vi "CTI_AOTF_GrabChannelFromGlobalVars.vi"(8 "error in":errorcluster) -> (0 "AOTF_LaserChannelWavelength":i32[](array[numeric]), 1 "AOTF_LaserChannelFixedwavelength":string[](array[string]), 2 "AOTF_LaserChannelPower":i16[](array[numeric]), 3 "AOTF_LaserChannelOnOff":bool[](array[boolean]), 4 "error out":errorcluster)   [LabVIEW 2011]
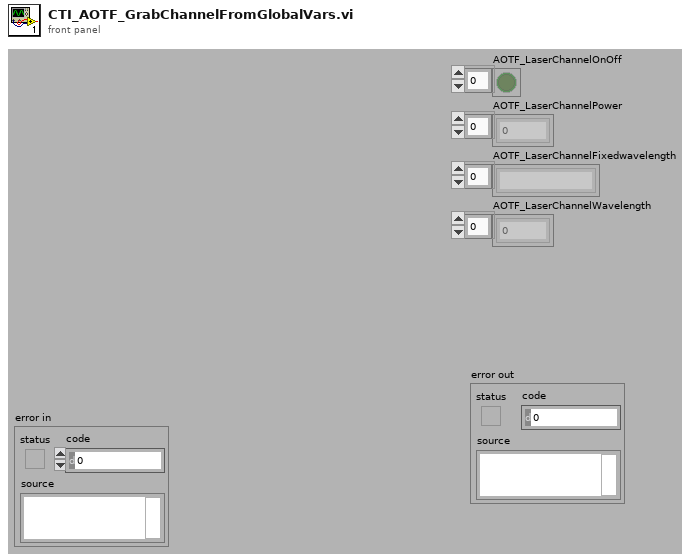
[diagram p1: front panel]
types:
  T1 = cluster{"1.LaserChannel ON/OFF":bool, "1.Laser Channel Power / [%]":i16, "1.Laser Channel Fixedwavelength":string, "1.Laser Channel Wavelength":i32, "Wavelength":enum16{"Fixed", "UserDefined"}}
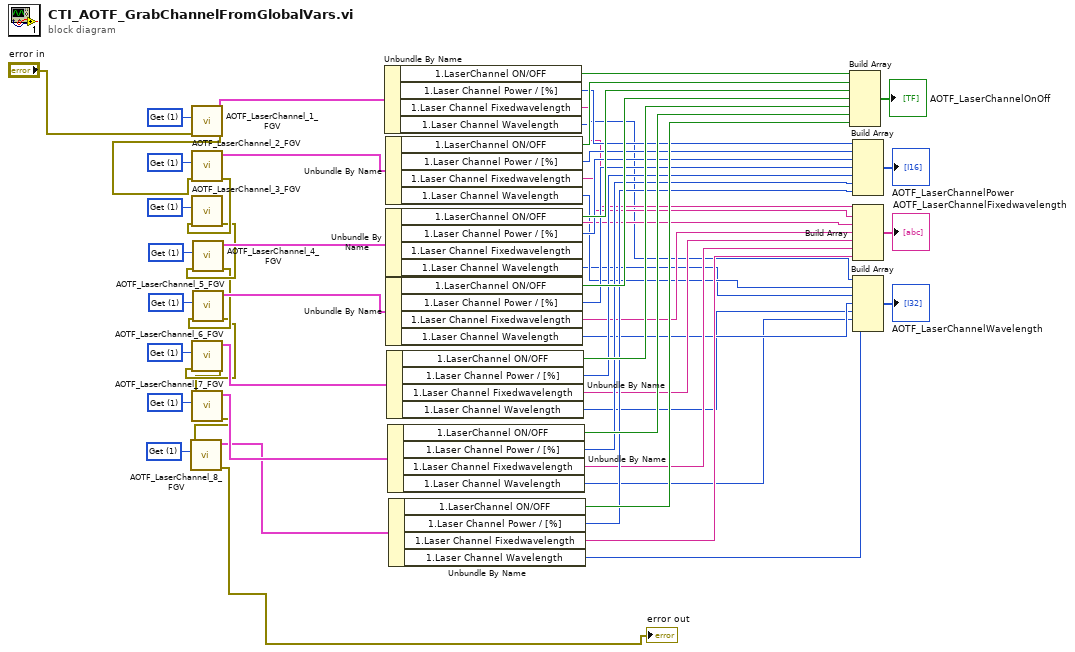
[diagram p0: block diagram]
diagram:
  w49 = u16 1 items=["Set", "Get"] ("Set_Get")
  w50 = u16 1 items=["Set", "Get"] ("Set_Get")
  w51 = u16 1 items=["Set", "Get"] ("Set_Get")
  w52 = u16 1 items=["Set", "Get"] ("Set_Get")
  w53 = u16 1 items=["Set", "Get"] ("Set_Get")
  w54 = u16 1 items=["Set", "Get"] ("Set_Get")
  w55 = u16 1 items=["Set", "Get"] ("Set_Get")
  w56 = u16 1 items=["Set", "Get"] ("Set_Get")
  n1 = call "AOTF_LaserChannel_1_FGV.vi"("error in"="error in", "Set_Get"=w56) -> ("error out"=w8:errorcluster, "LaserChannel_2_OUT"=w48:T1)  [unwired: 8 in]
  n2 = call "AOTF_LaserChannel_2_FGV.vi"("error in"=w8, "FGV_Control"=w55) -> ("error out"=w7:errorcluster, "LaserChannel_2_OUT"=w47:T1)  [unwired: 8 in]
  n3 = call "AOTF_LaserChannel_3_FGV.vi"("error in"=w7, "Set_Get"=w54) -> ("error out"=w6:errorcluster)  [unwired: 8 in, 1 out]
  n4 = call "AOTF_LaserChannel_4_FGV.vi"("error in"=w6, "Set_Get"=w53) -> ("error out"=w5:errorcluster, "LaserChannel_2_OUT"=w46:T1)  [unwired: 8 in]
  n5 = call "AOTF_LaserChannel_5_FGV.vi"("error in"=w5, "Set_Get"=w52) -> ("error out"=w4:errorcluster, "LaserChannel_2_OUT"=w45:T1)  [unwired: 8 in]
  n6 = call "AOTF_LaserChannel_6_FGV.vi"("error in"=w4, "Set_Get"=w51) -> ("error out"=w3:errorcluster, "LaserChannel_2_OUT"=w44:T1)  [unwired: 8 in]
  n7 = call "AOTF_LaserChannel_7_FGV.vi"("error in"=w3, "Set_Get"=w50) -> ("error out"=w2:errorcluster, "LaserChannel_2_OUT"=w43:T1)  [unwired: 8 in]
  n8 = call "AOTF_LaserChannel_8_FGV.vi"("error in"=w2, "Set_Get"=w49) -> ("error out"=→"error out":errorcluster, "LaserChannel_2_OUT"=w42:T1)  [unwired: 8 in]
  n9 = Unbundle By Name(w48) -> ("1.LaserChannel ON/OFF"=w41:bool, "1.Laser Channel Power / [%]"=w34:i16, "1.Laser Channel Fixedwavelength"=w27:string, "1.Laser Channel Wavelength"=w20:i32)
  n10 = Unbundle By Name(w47) -> ("1.LaserChannel ON/OFF"=w40:bool, "1.Laser Channel Power / [%]"=w33:i16, "1.Laser Channel Fixedwavelength"=w26:string, "1.Laser Channel Wavelength"=w19:i32)
  n11 = Unbundle By Name(w46) -> ("1.LaserChannel ON/OFF"=w39:bool, "1.Laser Channel Power / [%]"=w32:i16, "1.Laser Channel Fixedwavelength"=w25:string, "1.Laser Channel Wavelength"=w18:i32)
  n12 = Unbundle By Name(w45) -> ("1.LaserChannel ON/OFF"=w38:bool, "1.Laser Channel Power / [%]"=w31:i16, "1.Laser Channel Fixedwavelength"=w24:string, "1.Laser Channel Wavelength"=w17:i32)
  n13 = Unbundle By Name(w44) -> ("1.LaserChannel ON/OFF"=w37:bool, "1.Laser Channel Power / [%]"=w30:i16, "1.Laser Channel Fixedwavelength"=w23:string, "1.Laser Channel Wavelength"=w16:i32)
  n14 = Unbundle By Name(w43) -> ("1.LaserChannel ON/OFF"=w36:bool, "1.Laser Channel Power / [%]"=w29:i16, "1.Laser Channel Fixedwavelength"=w22:string, "1.Laser Channel Wavelength"=w15:i32)
  n15 = Unbundle By Name(w42) -> ("1.LaserChannel ON/OFF"=w35:bool, "1.Laser Channel Power / [%]"=w28:i16, "1.Laser Channel Fixedwavelength"=w21:string, "1.Laser Channel Wavelength"=w14:i32)
  n16 = Build Array(w41, w40, w39, w38, w37, w36, w35) -> (→"AOTF_LaserChannelOnOff":bool[])
  n17 = Build Array(w34, w33, w32, w31, w30, w29, w28) -> (→"AOTF_LaserChannelPower":i16[])
  n18 = Build Array(w27, w26, w25, w24, w23, w22, w21) -> (→"AOTF_LaserChannelFixedwavelength":string[])
  n19 = Build Array(w20, w19, w18, w17, w16, w15, w14) -> (→"AOTF_LaserChannelWavelength":i32[])
